vi "ListBox.vi"() -> ()   [LabVIEW 2015]
panel:
  in  "Item Names":string[](array[string])
  out "Status":i32(listbox)
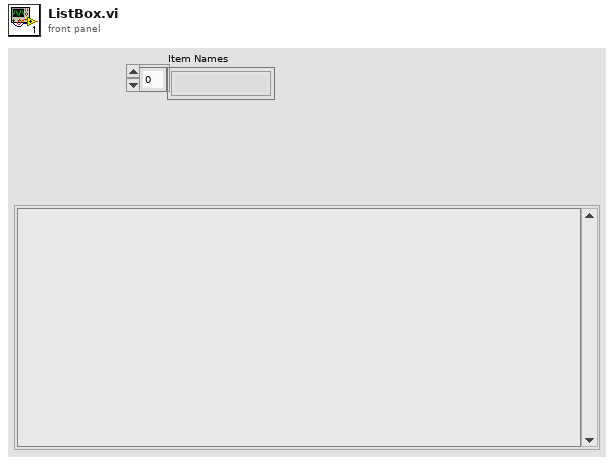
[diagram p1: front panel]
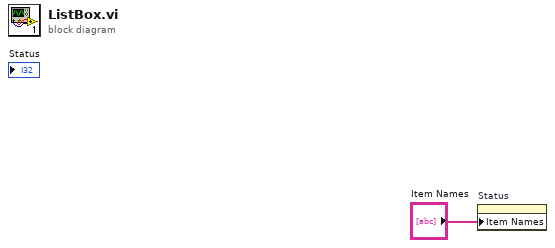
[diagram p0: block diagram]
diagram:
  n1 = property on="Status" class="LstBox (strict)"("Item Names"="Item Names") -> ()  [unwired: 2 in, 2 out]
